vi "Selection GUI.vi"() -> (0 "Continue Testing":bool, 1 "Total Cycles out":i32, 2 "DUTs.Cycle":bool[](array[boolean]), 3 "DUTs.SN":string[](array[string]), 4 "Start i":i32=1)   [LabVIEW 2014, in "NIAnalysis.lvlib"]
uses:
  NIAnalysis.lvlib
panel:
  in  "Start Cycle":i32=1 min=1
  in  "Total Cycles":i32=1000000
  in  "Start":bool
  in  "Enable 9":bool
  in  "DUT9 Serial Number":string
  in  "Enable 8":bool
  in  "DUT8 Serial Number":string
  in  "Enable 7":bool
  in  "DUT7 Serial Number":string
  in  "Enable 6":bool
  in  "DUT6 Serial Number":string
  in  "Enable 5":bool
  in  "DUT5 Serial Number":string
  in  "Enable 4":bool
  in  "DUT4 Serial Number":string
  in  "Enable 3":bool
  in  "DUT3 Serial Number":string
  in  "Enable 2":bool
  in  "DUT2 Serial Number":string
  in  "Enable 1":bool
  in  "DUT1 Serial Number":string
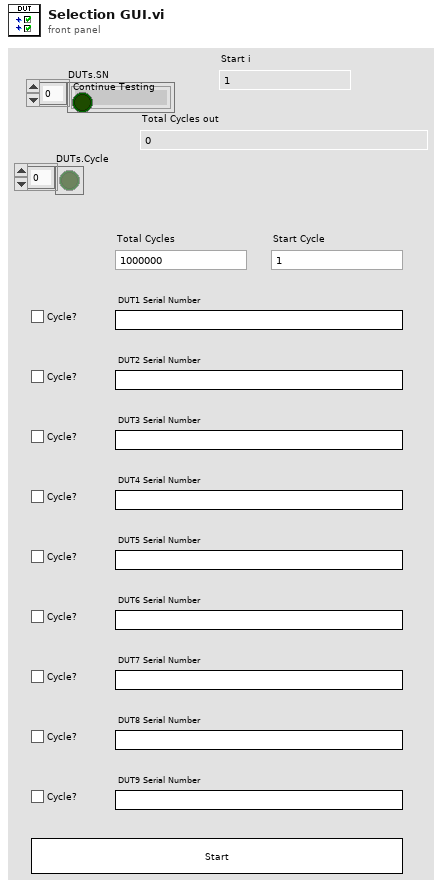
[diagram p1: front panel]
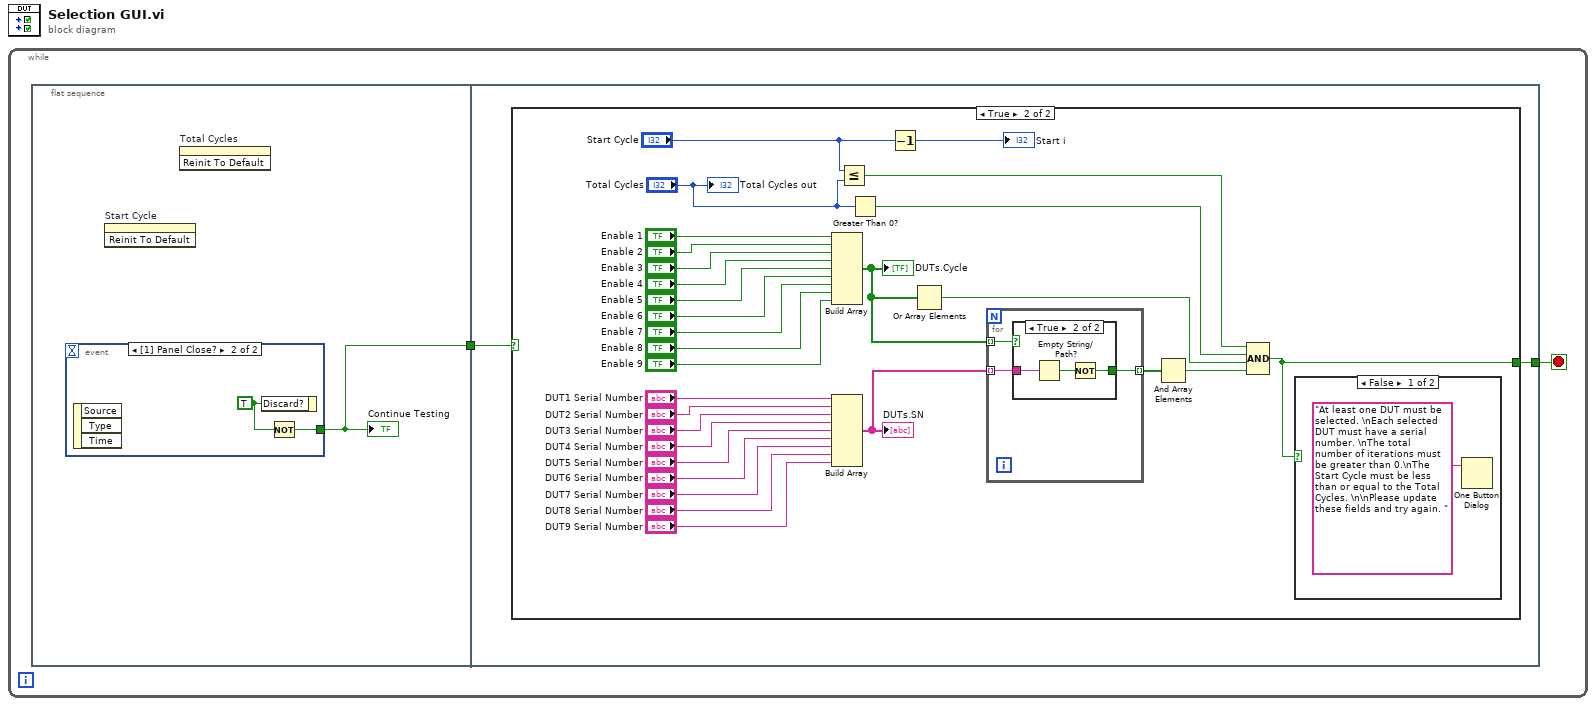
[diagram p0: block diagram]
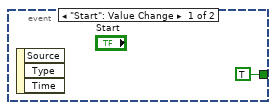
[diagram p2: hidden frame]
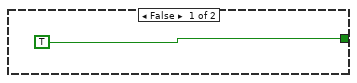
[diagram p3: hidden frame]
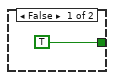
[diagram p5: hidden frame]
diagram:
  n1 = while {
    stop <- w2 stop-if-true
    n2 = flat-sequence {
      tunnel: [w3] -> w1
      tunnel: [w8] -> w2
      tunnel: w1 -> [w7]
      frame #0 {
        n3 = event shown="[1] Panel Close?" {
          selector: _ -> [_ _]
          dyn-events: _ -> [_ _]
          timeout: _ -> [_ _]
          tunnel: [TRUE ("Discard?") w5] -> w3
          event "Start": Value Change {
            n4 = event-data() -> ()  [unwired: 1 in, 3 out]
          }
          event Panel Close? {
            w6 = TRUE ("Discard?")
            n5 = event-data() -> ()  [unwired: 1 in, 3 out]
            n6 = event-data("Discard?"=w6) -> ()  [unwired: 1 in, 1 out]
            n7 = Not(x=w6) -> (.not. x?=w5:bool)
          }
        }
        "Continue Testing" <- w3
        n8 = invoke on="Start Cycle" class="DigNum (strict)" method="Reinit To Default"() -> ()  [unwired: 3 in, 3 out]
        n9 = invoke on="Total Cycles" class="DigNum (strict)" method="Reinit To Default"() -> ()  [unwired: 3 in, 3 out]
      }
      frame #1 {
        n10 = case shown="True" w7 {
          tunnel: [TRUE w16] -> w8
          frame False {
          }
          frame True {
            n11 = Build Array("Enable 1", "Enable 2", "Enable 3", "Enable 4", "Enable 5", "Enable 6", "Enable 7", "Enable 8", "Enable 9") -> (w15:bool[])
            "DUTs.Cycle" <- w15
            n12 = Build Array("DUT1 Serial Number", "DUT2 Serial Number", "DUT3 Serial Number", "DUT4 Serial Number", "DUT5 Serial Number", "DUT6 Serial Number", "DUT7 Serial Number", "DUT8 Serial Number", "DUT9 Serial Number") -> (w20:string[])
            "DUTs.SN" <- w20
            n13 = Less Or Equal?(x="Start Cycle", y="Total Cycles") -> (x <= y?=w10:bool)
            n14 = Greater Than 0?(x="Total Cycles") -> (x > 0?=w17:bool)
            n15 = Decrement(x="Start Cycle") -> (x-1=→"Start i":i32)
            n16 = Or Array Elements(Boolean array=w15) -> (logical OR=w14:bool)
            n17 = for {
              tunnel: w20 -> [w41] mode=indexing
              tunnel: w15 -> [w42] mode=indexing
              tunnel: [w40] -> w19 mode=indexing
              n18 = case shown="True" w42 {
                tunnel: w41 -> [_ w46]
                tunnel: [TRUE w44] -> w40
                frame False {
                }
                frame True {
                  n19 = Empty String/Path?(string/path=w46) -> (empty?=w45:bool)
                  n20 = Not(x=w45) -> (.not. x?=w44:bool)
                }
              }
            }
            n21 = And Array Elements(Boolean array=w19) -> (logical AND=w18:bool)
            n22 = Compound Arithmetic op=AND(w10, w17, w14, w18) -> (w16:bool)
            n23 = case shown="False" w16 {
              frame False {
                n24 = One Button Dialog(message="At least one DUT must be selected. \nEach selected DUT must have a serial number. \nThe total number of iterations must be greater than 0.\nThe Start Cycle must be less than or equal to the Total Cycles. \n\nPlease update these fields and try again. ") -> ()  [unwired: 1 in, 1 out]
              }
              frame True {
              }
            }
            "Total Cycles out" <- "Total Cycles"
          }
        }
      }
    }
  }
